vi "Launch Chart With Slider.vi"   [LabVIEW 2017]
uses:
  ExampleSimpleRootModel/SimpleRootModel.lvclass
  C:/Git/mva-framework/Framework/IModel/IModel/IModel.lvclass
  TwoPaneViewManager/TwoPaneViewManager.lvclass
  C:/Git/mva-framework/Framework/IViewManager/IViewManager/IViewManager.lvclass
  C:/Git/mva-framework/Framework/IViewable/IViewable/IViewable.lvclass
  SimpleViewModel/SimpleViewModel.lvclass
  C:/Git/mva-framework/Framework/IViewModel/IViewModel/IViewModel.lvclass
  C:/Program Files (x86)/National Instruments/LabVIEW 2017/vi.lib/ActorFramework/Actor/Actor.lvclass
  Source/Framework/Mediator/Mediator/Mediator.lvclass
  C:/Git/mva-framework/Framework/IMediator/IMediator/IMediator.lvclass
  Source/Framework/Mediator/MediatorBusMonitor/MediatorBusMonitor.lvclass
  C:/Git/mva-framework/Framework/IMediator/IMediatorBusMonitor/MediatorBusMonitor/IMediatorBusMonitor.lvclass
  <vilib>/ActorFramework/Message Enqueuer/Message Priority.ctl
  Source/Framework/IViewable/IViewable/View Position Enum.ctl
  SimpleChart/SimpleChart.lvclass
  VerticalSlide/VerticalSlide.lvclass
  ExampleSimpleRootModel/SimpleRootModel.lvclass/SimpleRootModel.ctl
  Source/Framework/IViewManager/IViewManager Messages/Launch Nested Views Msg/Launch Nested Views Msg.lvclass/Launch Nested Views Msg.ctl
  Source/Framework/IViewManager/IViewManager/IViewManager.lvclass/IViewManager.ctl
  Source/Framework/IMediator/IMediator/IMediator.lvclass/IMediator.ctl
  Source/Framework/IViewModel/IViewModel/IViewModel.lvclass/IViewModel.ctl
  Source/Framework/IViewable/IViewable Messages/Open Front Panel Msg/Open Front Panel Msg.lvclass/Open Front Panel Msg.ctl
  <vilib>/ActorFramework/Message Enqueuer/Message Enqueuer.lvclass/Message Enqueuer.ctl
  Source/Framework/IViewManager/IViewManager Messages/Launch Nested Views Msg/Pack Launch Nested Views Msg.vi
  Source/Framework/IViewManager/IViewManager/Write Startup Launch Nested Views Msg.vi
  <vilib>/ActorFramework/Message Enqueuer/Enqueue.vi
  Source/Framework/IViewModel/IViewModel/IViewModel.lvclass
  Source/Framework/IViewable/IViewable Messages/Open Front Panel Msg/Open Front Panel Msg.lvclass
  C:/Program Files (x86)/National Instruments/LabVIEW 2017/vi.lib/ActorFramework/Message/Message.lvclass
  <vilib>/ActorFramework/Message Priority Queue/Priority Enqueue.vi
  Source/Framework/IViewManager/IViewManager Messages/Launch Nested Views Msg/Launch Nested Views Msg.lvclass
  Source/Framework/IViewable/IApplicationStyle/IApplicationStyle.lvclass
  <vilib>/ActorFramework/Actor/Actor.lvclass
  Source/Framework/IMediator/IMediator/IMediator.lvclass
  <vilib>/ActorFramework/Message Enqueuer/Message Enqueuer.lvclass
  Source/Framework/IViewable/IViewable/IViewable.lvclass
  Source/Framework/IViewManager/IViewManager/IViewManager.lvclass
panel:
  # "This example launches a two-pane MVA application"
types:
  T1 = typedef "IViewable.lvlib/IViewable.lvclass/View Position Enum.ctl" = enum16{"Centered", "Maximized", "Minimized", "Custom", "Unchanged"}
  T2 = typedef "Actor Framework.lvlib/Message Enqueuer.lvclass/Message Priority.ctl" = enum16{"Low", "Normal", "High"}
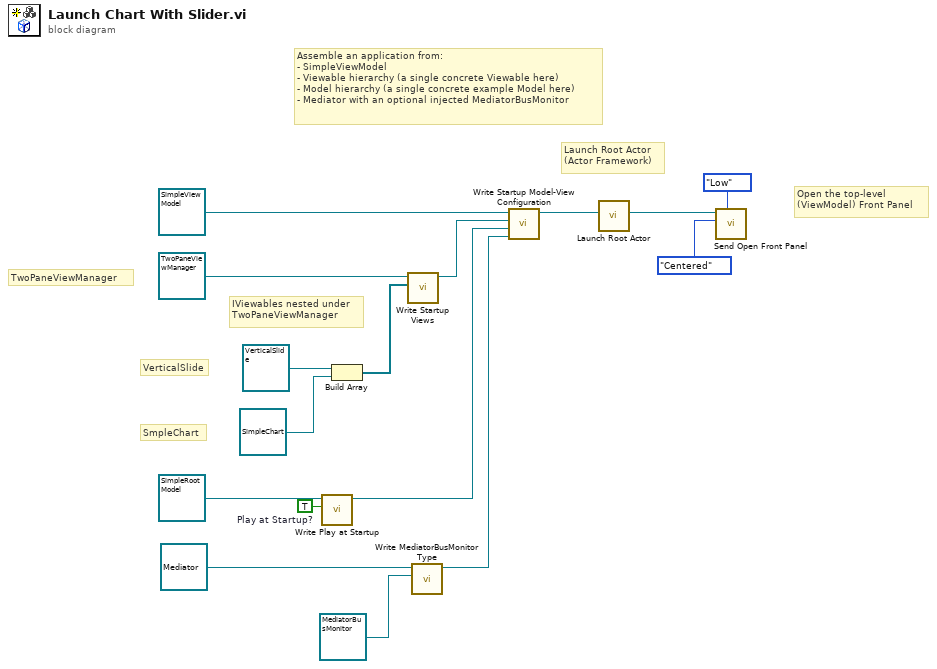
[diagram p0: block diagram]
diagram:
  w1 = TRUE  # Play at Startup?
  # "SmpleChart"
  # "VerticalSlide"
  # "IViewables nested under \nTwoPaneViewManager"
  # "TwoPaneViewManager"
  # "Open the top-level\n(ViewModel) Front Panel"
  # "Launch Root Actor\n(Actor Framework)"
  # "Assemble an application from:\n- SimpleViewModel\n- Viewable hierarchy (a single concrete Viewable here)\n- Model hierarchy (a single concrete example Model here)\n- Mediator with an optional injected MediatorBusMonitor"
  n1 = call "Write Play at Startup.vi"("Play at Startup?"=w1, "SimpleRootModel in"=refnum<class "SimpleRootModel.lvclass"> refnum ("MVAExamples.lvlib:SimpleRootModel.lvclass")) -> ("SimpleRootModel out"=w2:refnum<class "SimpleRootModel.lvclass">)  [unwired: 9 in]
  n2 = Build Array(refnum<class "VerticalSlide.lvclass"> refnum ("MVAExamples.lvlib:VerticalSlide.lvclass"), refnum<class "SimpleChart.lvclass"> refnum ("MVAExamples.lvlib:SimpleChart.lvclass")) -> (w3:refnum<class "IViewable.lvclass">[])
  n3 = call "Write Startup Views.vi"("Startup Views"=w3, "IViewManager in"=refnum<class "TwoPaneViewManager.lvclass"> refnum ("MVAExamples.lvlib:TwoPaneViewManager.lvclass")) -> ("IViewManager out"=w6:refnum<class "TwoPaneViewManager.lvclass">)  [unwired: 9 in]
  n4 = call "Write MediatorBusMonitor Type.vi"("MediatorBusMonitor (Type)"=refnum<class "MediatorBusMonitor.lvclass"> refnum ("Mediator.lvlib:MediatorBusMonitor.lvclass"), "IMediator in"=refnum<class "Mediator.lvclass"> refnum ("Mediator.lvlib:Mediator.lvclass")) -> ("IMediator out"=w11:refnum<class "Mediator.lvclass">)  [unwired: 9 in]
  n5 = call "Write Startup Model-View Configuration.vi"("Mediator Type"=w11, "Model Type"=w2, "Startup View Configuration"=w6, "IViewModel In"=refnum<class "SimpleViewModel.lvclass"> refnum ("MVAExamples.lvlib:SimpleViewModel.lvclass")) -> ("IViewModel Out"=w10:refnum<class "SimpleViewModel.lvclass">)  [unwired: 7 in]
  n6 = call <vilib>:"Launch Root Actor.vi"("Actor"=w10) -> ("Actor's Enqueuer"=w9:refnum<class "Message Enqueuer.lvclass">)  [unwired: 9 in, 1 out]
  n7 = call "Send Open Front Panel.vi"("Message Priority (Normal)"=Message_Priority."Low", "Position"=View_Position_Enum."Centered", "Message Enqueuer"=w9) -> ()  [unwired: 7 in, 2 out]
